vi "IndentItem__slk_tc.vi"(0 "tree control in":refnum<class "TreeControl.lvclass">, 5 "indent tag (current tag)":string, 11 "error in (no error)":errorcluster) -> (4 "tree control out":refnum<class "TreeControl.lvclass">, 15 "error out":errorcluster)   [LabVIEW 2020, in "TreeControl.lvclass"]
doc: "Takes the input tag item and places it along with its children as a child family of its current topmost sibling. Ignores the indent command if there is no current sibling to indent under."
uses:
  Library/TreeControl.lvclass
  Library/TreeControl.lvclass/TreeControl.ctl
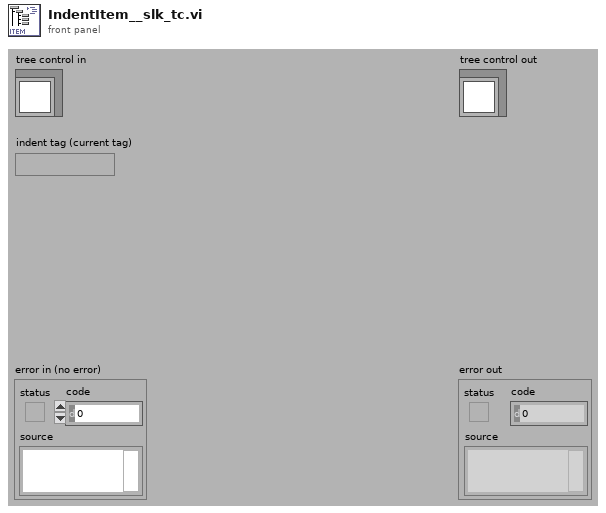
[diagram p1: front panel]
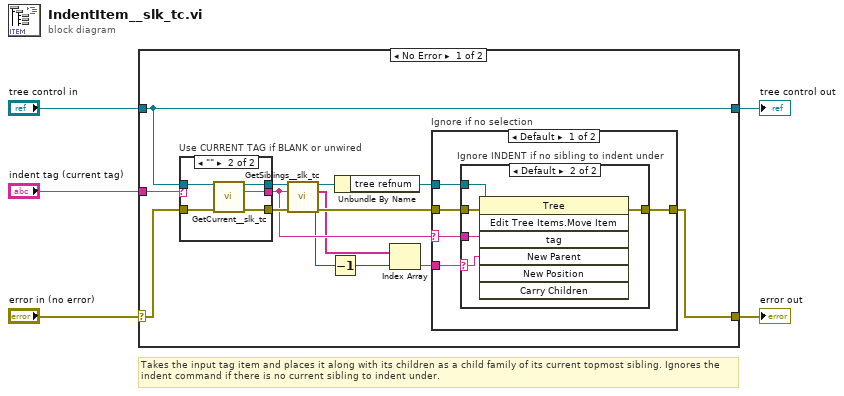
[diagram p0: block diagram]
diagram:
  # "Takes the input tag item and places it along with its children as a child family of its current topmost sibling. Ignores the indent command if there is no current sibling to indent under."
  n1 = case shown="No Error" "error in (no error)" {
    selector: "error in (no error)" -> [w9 w41]
    tunnel: [w8 w41] -> w4
    tunnel: [w18 w40] -> w2
    tunnel: "tree control in" -> [w18 w40]
    tunnel: "indent tag (current tag)" -> [w19 _]
    frame No Error {
      n2 = case "Use CURRENT TAG if BLANK or unwired" shown="\"\"" w19 {
        selector: w19 -> [w34 _]
        tunnel: [w34 w39] -> w15
        tunnel: w18 -> [w32 w38]
        tunnel: w9 -> [w33 w37]
        tunnel: [w33 w36] -> w16
        tunnel: [w32 w35] -> w17
        frame Default {
        }
        frame "" {
          n3 = call "GetCurrent__slk_tc.vi"("tree control in"=w38, "error in (no error)"=w37) -> ("tree control out"=w35:refnum<class "TreeControl.lvclass">, "current tag"=w39:string, "error out"=w36:errorcluster)  [unwired: 1 in, 10 out]
        }
      }
      n4 = call "GetSiblings__slk_tc.vi"("tree control in"=w17, "input tag (current tag)"=w15, "error in (no error)"=w16) -> ("tree control out"=w14:refnum<class "TreeControl.lvclass">, "sibling tags"=w11:string[], "input tag index"=w7:i32, "error out"=w12:errorcluster)  [unwired: 9 out]
      n5 = Decrement(x=w7) -> (x-1=w6:i32)
      n6 = Unbundle By Name(w14) -> ("tree refnum"=w13:refnum<vi>)
      n7 = Index Array(array=w11, index=w6) -> (element=w10:string)
      n8 = case "Ignore if no selection" shown="Default" w15 {
        selector: w15 -> [w22 _]
        tunnel: w13 -> [w21 _]
        tunnel: w12 -> [w24 w31]
        tunnel: w10 -> [w23 _]
        tunnel: [w20 w31] -> w8
        frame Default {
          n9 = case "Ignore INDENT if no sibling to indent under" shown="Default" w23 {
            selector: w23 -> [_ w26]
            tunnel: w24 -> [w25 w30]
            tunnel: w22 -> [_ w29]
            tunnel: [w25 w28] -> w20
            tunnel: w21 -> [_ w27]
            frame "" {
            }
            frame Default {
              n10 = invoke class="Tree" method="Edit Tree Items.Move Item"(reference=w27, error in=w30, "tag"=w29, "New Parent"=w26) -> (error out=w28:errorcluster)  [unwired: 3 in, 6 out]
            }
          }
        }
        frame "" {
        }
      }
    }
    frame Error {
    }
  }
  "error out" <- w4
  "tree control out" <- w2
